vi "Check if configuration files exist.vi"(8 "error in (no error)":errorcluster, 11 "RSABase in":refnum<class "RSA.lvclass">) -> (0 "error out":errorcluster, 2 "configuration file exists?":bool, 3 "RSABase out":refnum<class "RSA.lvclass">)   [LabVIEW 2012, in "RSA.lvclass"]
doc: "Checks whether all required configuration files for the component exist."
uses:
  RSA.lvclass
  <vilib>/Distrio/Murmex/Murmex/Murmex.lvclass
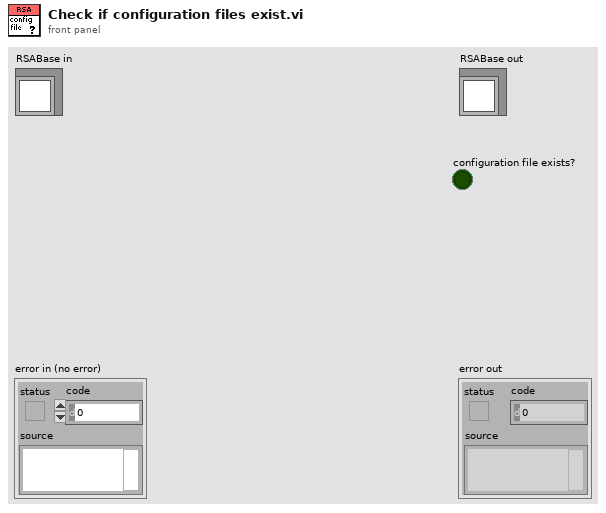
[diagram p1: front panel]
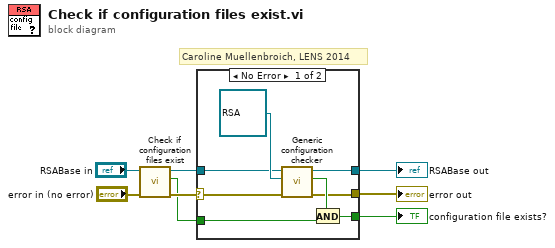
[diagram p0: block diagram]
diagram:
  # "Caroline Muellenbroich, LENS 2014"
  n1 = call-parent "Check if configuration files exist.vi"("error in (no error)"="error in (no error)", "MurmexBase in"="RSABase in") -> ("error out"=w6:errorcluster, "configuration file exists?"=w3:bool, "MurmexBase out"=w5:refnum<class "RSA.lvclass">)  [unwired: 7 in]
  n2 = case shown="No Error" w6 {
    selector: w6 -> [w13 w18]
    tunnel: w5 -> [w14 w19]
    tunnel: [w12 w18] -> w4
    tunnel: w3 -> [w11 w17]
    tunnel: [w10 w17] -> w2
    tunnel: [w9 w19] -> w1
    frame No Error {
      n3 = call <vilib>:"Generic configuration checker.vi"("error in (no error)"=w13, "inheritance level"=refnum<class "RSA.lvclass"> refnum ("RSA"), "Murmex in"=w14) -> ("error out"=w12:errorcluster, "configuration file exists?"=w16:bool, "Murmex out"=w9:refnum<class "RSA.lvclass">)  [unwired: 6 in]
      n4 = And(x=w16, y=w11) -> (x .and. y?=w10:bool)
    }
    frame Error {
    }
  }
  "error out" <- w4
  "RSABase out" <- w1
  "configuration file exists?" <- w2
